vi "Tosca-Remap Adaptation Variables.vi"(0 "Adapt In":T1, 11 "error in (no error)":errorcluster, 12 "AO Name Map":cluster{"old":string[], "new":string[]}) -> (4 "Adapt Out":T1, 15 "error out":errorcluster)   [LabVIEW 2015]
uses:
  Typedefs/Tosca-Adapt.ctl
  Typedefs/Tosca-Adaptive Track.ctl
  Typedefs/Tosca-Simple Variable.ctl
  Adaptation VIs/Tosca-Adapt Threshold Metric.ctl
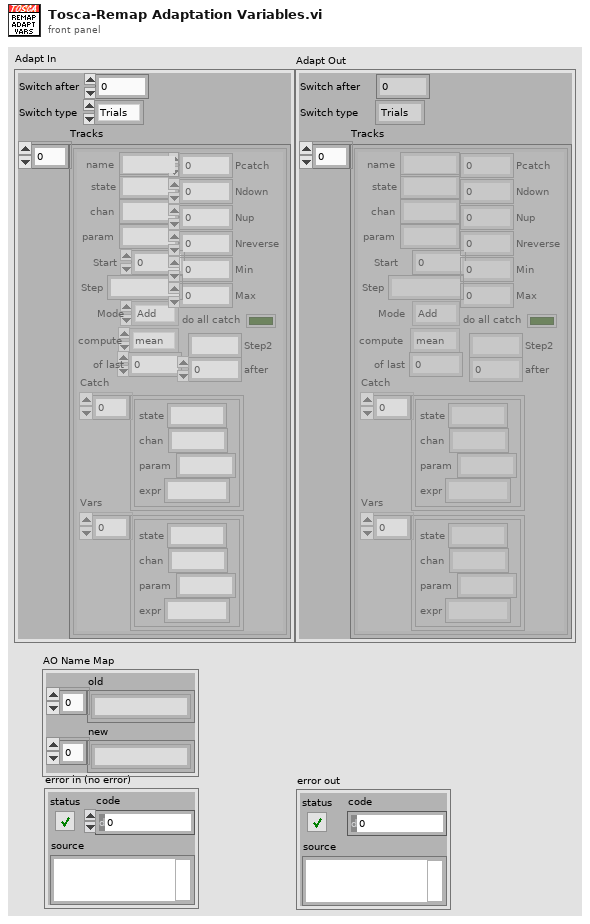
[diagram p1: front panel]
types:
  T1 = typedef "Tosca-Adapt.ctl" = cluster{"Switch after":i32, "Switch type":enum16{"Trials", "Reversals"}, "Tracks":T2[]}
  T2 = typedef "Tosca-Adaptive Track.ctl" = cluster{"state":string, "chan":string, "param":string, "Start":dbl, "Step":string, "Mode":enum16{"Add", "Multiply"}, "Pcatch":dbl, "Ndown":i32, "Nup":i32, "Nreverse":i32, "Min":dbl, "Max":dbl, "Catch":T3[], "do all catch":bool, "name":string, "Vars":T3[], "compute":T4, "of last":i32, "Step2":string, "after":i32}
  T3 = typedef "Tosca-Simple Variable.ctl" = cluster{"state":string, "chan":string, "param":string, "expr":string}
  T4 = typedef "Tosca-Adapt Threshold Metric.ctl" = enum16{"mean", "median"}
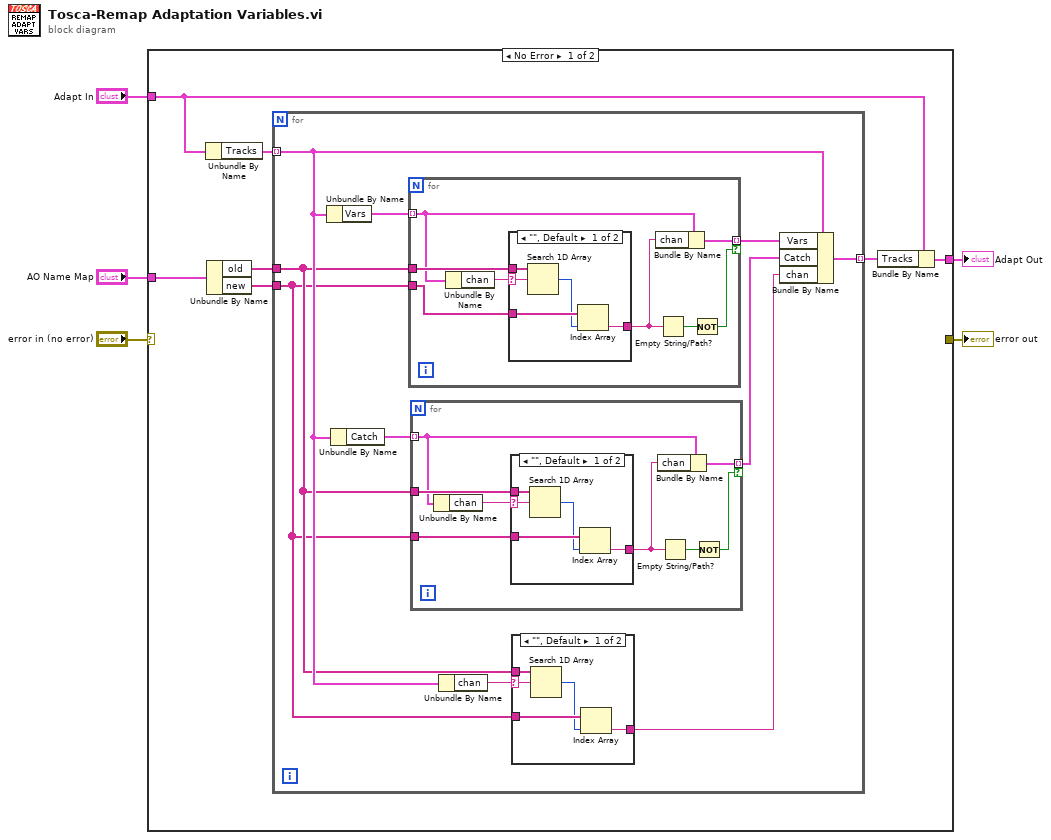
[diagram p0: block diagram]
diagram:
  n1 = case shown="No Error" "error in (no error)" {
    selector: "error in (no error)" -> [_ w58]
    tunnel: "AO Name Map" -> [w12 _]
    tunnel: [w6 w57] -> w1
    tunnel: [_ w58] -> w3
    tunnel: "Adapt In" -> [w7 w57]
    frame No Error {
      n2 = Unbundle By Name(w7) -> ("Tracks"=w11:T2[])
      n3 = Unbundle By Name(w12) -> ("old"=w10:string[], "new"=w9:string[])
      n4 = for {
        tunnel: w11 -> [w16] mode=indexing
        tunnel: w10 -> [w15]
        tunnel: w9 -> [w14]
        tunnel: [w21] -> w8 mode=indexing
        n5 = Unbundle By Name(w16) -> ("Vars"=w22:T3[])
        n6 = Unbundle By Name(w16) -> ("Catch"=w19:T3[])
        n7 = for {
          tunnel: w22 -> [w42] mode=indexing
          tunnel: w15 -> [w44]
          tunnel: w14 -> [w43]
          tunnel: [w41] -> w20 mode=indexing if=w38
          n8 = Unbundle By Name(w42) -> ("chan"=w37:string)
          n9 = case shown="\"\", Default" w37 {
            selector: w37 -> [w45 w50]
            tunnel: w44 -> [w49 _]
            tunnel: w43 -> [w48 _]
            tunnel: [w46 w50] -> w40
            frame "", Default {
              n10 = Search 1D Array(1D array=w49, element=w45) -> (index of element=w47:i32)  [unwired: 1 in]
              n11 = Index Array(array=w48, index=w47) -> (element=w46:string)
            }
            frame "---" {
            }
          }
          n12 = Bundle By Name(cluster=w42, "chan"=w40) -> (w41:T3)
          n13 = Empty String/Path?(string/path=w40) -> (empty?=w39:bool)
          n14 = Not(x=w39) -> (.not. x?=w38:bool)
        }
        n15 = for {
          tunnel: w19 -> [w28] mode=indexing
          tunnel: w15 -> [w30]
          tunnel: w14 -> [w29]
          tunnel: [w27] -> w18 mode=indexing if=w24
          n16 = Unbundle By Name(w28) -> ("chan"=w23:string)
          n17 = case shown="\"\", Default" w23 {
            selector: w23 -> [w31 w36]
            tunnel: w30 -> [w35 _]
            tunnel: w29 -> [w34 _]
            tunnel: [w32 w36] -> w26
            frame "", Default {
              n18 = Search 1D Array(1D array=w35, element=w31) -> (index of element=w33:i32)  [unwired: 1 in]
              n19 = Index Array(array=w34, index=w33) -> (element=w32:string)
            }
            frame "---" {
            }
          }
          n20 = Bundle By Name(cluster=w28, "chan"=w26) -> (w27:T3)
          n21 = Empty String/Path?(string/path=w26) -> (empty?=w25:bool)
          n22 = Not(x=w25) -> (.not. x?=w24:bool)
        }
        n23 = Unbundle By Name(w16) -> ("chan"=w17:string)
        n24 = case shown="\"\", Default" w17 {
          selector: w17 -> [w51 w56]
          tunnel: w15 -> [w55 _]
          tunnel: w14 -> [w54 _]
          tunnel: [w52 w56] -> w13
          frame "", Default {
            n25 = Search 1D Array(1D array=w55, element=w51) -> (index of element=w53:i32)  [unwired: 1 in]
            n26 = Index Array(array=w54, index=w53) -> (element=w52:string)
          }
          frame "---" {
          }
        }
        n27 = Bundle By Name(cluster=w16, "Vars"=w20, "Catch"=w18, "chan"=w13) -> (w21:T2)
      }
      n28 = Bundle By Name(cluster=w7, "Tracks"=w8) -> (w6:T1)
    }
    frame Error {
    }
  }
  "error out" <- w3
  "Adapt Out" <- w1
